vi "Get Log Control Reference.vi"(8 "エラー入力 (エラーなし)":errorcluster, 11 "Log Control  Name":string) -> (0 "エラー出力":errorcluster, 3 "Referece to Log Control":refnum<vi>)   [LabVIEW 2014]
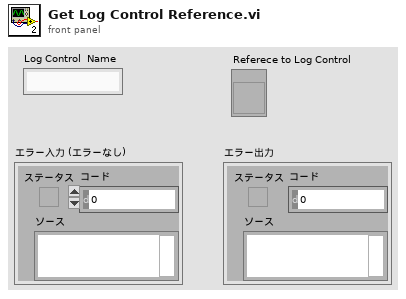
[diagram p1: front panel]
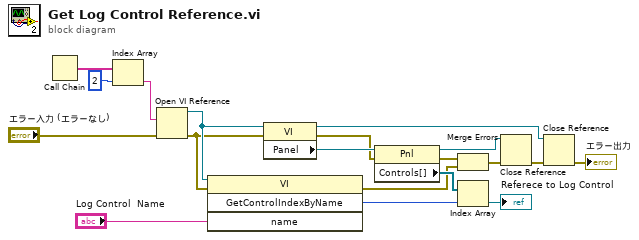
[diagram p0: block diagram]
diagram:
  n1 = Call Chain() -> (call chain=w5:string[])
  n2 = Index Array(array=w5, index=2 ("Žw•W")) -> (element=w3:string)
  n3 = Open VI Reference(vi path=w3, error in (no error)="エラー入力 (エラーなし)") -> (vi reference=w15:refnum<vi>, error out=w11:errorcluster)  [unwired: 4 in]
  n4 = invoke class="VI" method="GetControlIndexByName"(reference=w15, error in=w11, "name"="Log Control  Name") -> (error out=w6:errorcluster, "GetControlIndexByName"=w1:i32)  [unwired: 1 in, 2 out]
  n5 = property class="VI"(reference=w15, error in=w11) -> (reference out=w9:refnum<vi>, error out=w12:errorcluster, "Panel"=w16:refnum<vi>)
  n6 = property class="Pnl"(reference=w16, error in=w12) -> (reference out=w10:refnum<vi>, error out=w7:errorcluster, "Controls[]"=w13:refnum<vi>[])
  n7 = Merge Errors(w7, w6) -> (w17:errorcluster)
  n8 = Index Array(array=w13, index=w1) -> (element=→"Referece to Log Control":refnum<vi>)
  n9 = Close Reference(reference=w10, error in (no error)=w17) -> (error out=w8:errorcluster)
  n10 = Close Reference(reference=w9, error in (no error)=w8) -> (error out=→"エラー出力":errorcluster)
